vi "Launch Default MainPane Actor.vi"(8 "error in (no error)":errorcluster, 9 "Stop Existing? (T)":bool=TRUE, 11 "MainController in":refnum<class "MainController.lvclass">) -> (0 "error out":errorcluster, 2 "Enqueuer":refnum<class "Message Enqueuer.lvclass">, 3 "MainController out":refnum<class "MainController.lvclass">)   [LabVIEW 2012, in "Win8uiFramework.lvlib" / "MainController.lvclass"]
uses:
  MainController.lvclass
  <vilib>/ActorFramework/Message Enqueuer/Message Enqueuer.lvclass
  MainController.lvclass/MainController.ctl
  <vilib>/ActorFramework/Actor/Actor.lvclass/Actor.ctl
  <vilib>/ActorFramework/Message Enqueuer/Message Enqueuer.lvclass/Message Enqueuer.ctl
  Read Default MainPane Actor.vi
  Read MainPane Enqueuer.vi
  Write MainPane Enqueuer.vi
  <vilib>/ActorFramework/Message Enqueuer/Enqueue.vi
  <vilib>/ActorFramework/Message Enqueuer/Init from Existing Queue.vi
  <vilib>/ActorFramework/Message Priority Queue/Priority Enqueue.vi
  ViewableActor.lvclass
  <vilib>/ActorFramework/Stop Msg/Stop Msg.lvclass
  <vilib>/ActorFramework/Actor/Actor.lvclass
  Win8uiFramework.lvlib
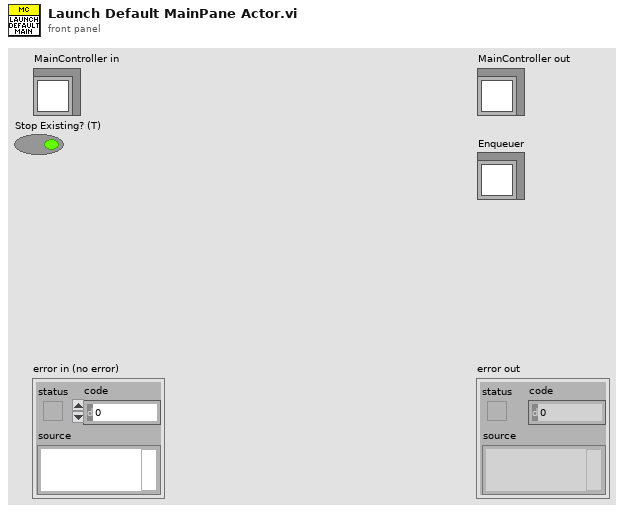
[diagram p1: front panel]
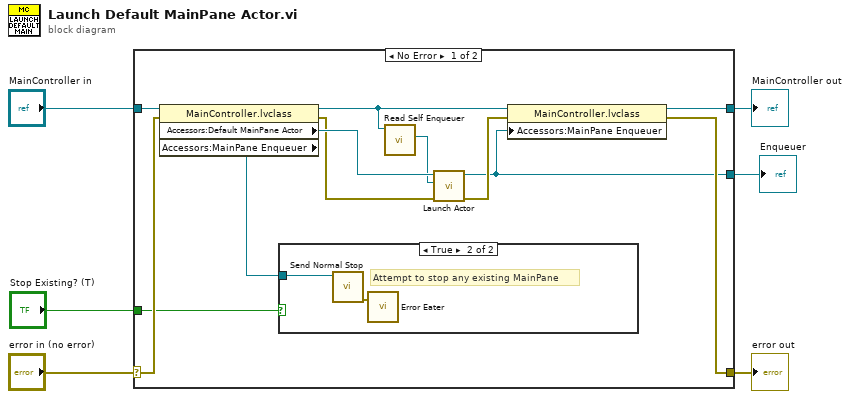
[diagram p0: block diagram]
diagram:
  n1 = case shown="No Error" "error in (no error)" {
    selector: "error in (no error)" -> [w11 w22]
    tunnel: [w10 w22] -> w5
    tunnel: [w17 w21] -> w3
    tunnel: "MainController in" -> [w18 w21]
    tunnel: [w9 _] -> w2
    tunnel: "Stop Existing? (T)" -> [w7 _]
    frame No Error {
      n2 = property class="MainController.lvclass"(reference=w18, error in=w11) -> (reference out=w15:refnum<class "MainController.lvclass">, error out=w13:errorcluster, "Accessors:Default MainPane Actor"=w16:refnum<class "ViewableActor.lvclass">, "Accessors:MainPane Enqueuer"=w8:refnum<class "Message Enqueuer.lvclass">)
      n3 = case shown="True" w7 {
        tunnel: w8 -> [_ w19]
        frame False {
        }
        frame True {
          # "Attempt to stop any existing MainPane"
          n4 = call <vilib>:"Send Normal Stop.vi"("Message Enqueuer"=w19) -> ("error out"=w20:errorcluster)  [unwired: 10 in]
          n5 = call "Error Eater.vi"("error in (no error)"=w20) -> ()  [unwired: 2 in]
        }
      }
      n6 = call <vilib>:"Read Self Enqueuer.vi"("Actor"=w15) -> ("Self Enqueuer"=w14:refnum<class "Message Enqueuer.lvclass">)  [unwired: 10 in]
      n7 = call <vilib>:"Launch Actor.vi"("error in (no error)"=w13, "Actor-to-Caller Enqueuer"=w14, "Actor"=w16) -> ("error out"=w12:errorcluster, "Caller-To-Actor Enqueuer"=w9:refnum<class "Message Enqueuer.lvclass">)  [unwired: 7 in]
      n8 = property class="MainController.lvclass"(reference=w15, error in=w12, "Accessors:MainPane Enqueuer"=w9) -> (reference out=w17:refnum<class "MainController.lvclass">, error out=w10:errorcluster)
    }
    frame Error {
    }
  }
  "error out" <- w5
  "MainController out" <- w3
  "Enqueuer" <- w2
